vi "add channel to configuration.vi"(8 "error in":errorcluster, 10 "channel":refnum<class "TBM channel.lvclass">, 11 "Scaling configuration in":refnum<class "Scaling configuration.lvclass">) -> (0 "error out":errorcluster, 3 "Scaling configuration out":refnum<class "Scaling configuration.lvclass">)   [LabVIEW 2013, in "Scaling configuration.lvclass"]
uses:
  Scaling configuration.lvclass
  <vilib>/NI/Tag Bus Module Framework/channel/TBM channel.lvclass
  <vilib>/NI/Tag Bus/tag/tag descriptor.lvclass
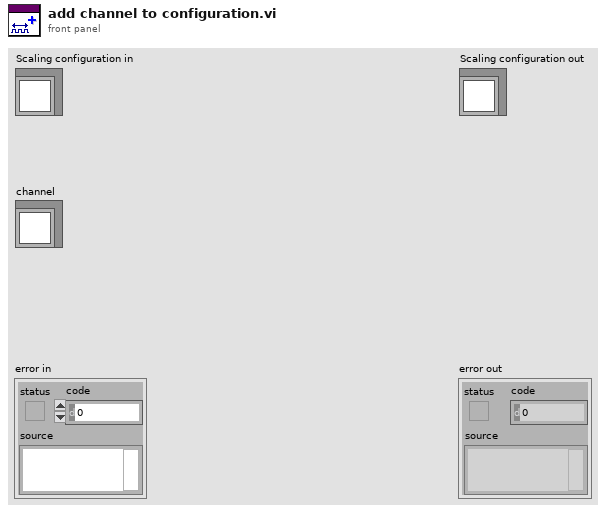
[diagram p1: front panel]
types:
  T1 = typedef "Scaling configuration.lvclass/scale data types.ctl" = enum16{"Double", "Single", "I64", "I32", "I16", "I8", "U64", "U32", "U16", "U8"}
  T2 = cluster{"input channel":refnum<class "TBM channel.lvclass">, "output channel":refnum<class "TBM channel.lvclass">, "input data type":T1, "output data type":T1}[][]
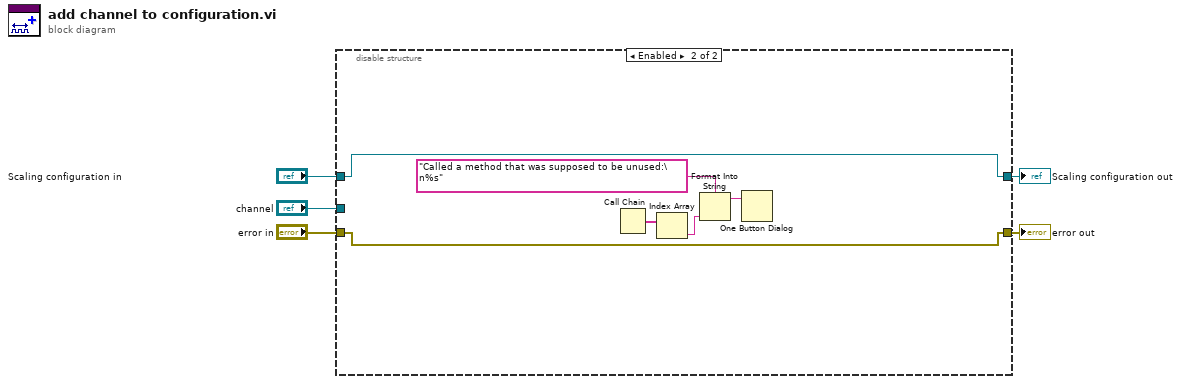
[diagram p0: block diagram]
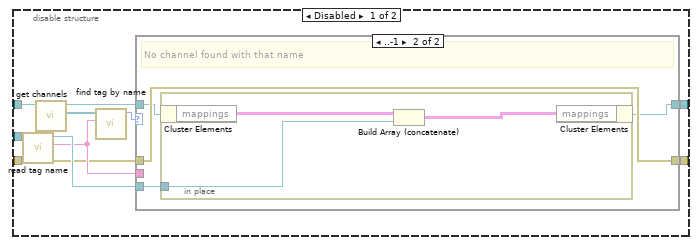
[diagram p2: hidden frame]
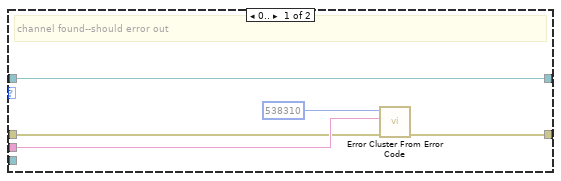
[diagram p3: hidden frame]
diagram:
  n1 = disable-structure shown="Enabled" {
    disable-tunnel: "channel" -> [w14 _]
    disable-tunnel: [w13 w29] -> w4
    disable-tunnel: [w12 w30] -> w3
    disable-tunnel: "Scaling configuration in" -> [w11 w30]
    disable-tunnel: "error in" -> [w6 w29]
    frame Disabled {
      n2 = call <vilib>:"read tag name.vi"("error in"=w6, "system tag in"=w14) -> ("error out"=w7:errorcluster, "name"=w8:string, "system tag out"=w15:refnum<class "TBM channel.lvclass">)  [unwired: 7 in]
      n3 = call-dynamic "get channels.vi"("Scaling configuration in"=w11) -> ("channels"=w10:refnum<class "TBM channel.lvclass">[], "Scaling configuration out"=w16:refnum<class "Scaling configuration.lvclass">)  [unwired: 9 in]
      n4 = call <vilib>:"find tag by name.vi"("name"=w8, "tags in"=w10) -> ("index"=w9:i32)  [unwired: 9 in]
      n5 = case shown="..-1" w9 {
        tunnel: [w21 w24] -> w13
        tunnel: w8 -> [w19 _]
        tunnel: w7 -> [w18 w24]
        tunnel: w16 -> [w17 w23]
        tunnel: w15 -> [_ w25]
        tunnel: [w17 w22] -> w12
        frame 0.. {
          # "channel found--should error out"
          n6 = call <vilib>:"Error Cluster From Error Code.vi"("error in (no error)"=w18, "error message (\"\")"=w19, "error code (0)"=538310) -> ("error out"=w21:errorcluster)  [unwired: 6 in]
        }
        frame ..-1 {
          # "No channel found with that name"
          n7 = in-place {
            in-place-border: w25 -> [w28]
            n8 = in-place-cluster #1(w23) -> ("mappings"=w26:T2)
            n9 = Build Array (concatenate)(w26, w28) -> (w27:T2)
            n10 = in-place-cluster #1("mappings"=w27) -> (w22:refnum<class "Scaling configuration.lvclass">)
          }
        }
      }
    }
    frame Enabled {
      n11 = Call Chain() -> (call chain=w34:string[])
      n12 = Index Array(array=w34) -> (element=w33:string)  [unwired: 1 in]
      n13 = Format Into String(format string="Called a method that was supposed to be unused:\n%s", w33) -> (resulting string=w31:string)  [unwired: 2 in, 1 out]
      n14 = One Button Dialog(message=w31) -> ()  [unwired: 1 in, 1 out]
    }
  }
  "error out" <- w4
  "Scaling configuration out" <- w3
